vi "Read Cameras.vi"(8 "error in (no error)":errorcluster, 11 "Gantry Class in":refnum<class "Gantry Class.lvclass">) -> (0 "error out":errorcluster, 2 "Cameras":T1[](array[typedef]), 3 "Gantry Class out":refnum<class "Gantry Class.lvclass">)   [LabVIEW 2011, in "Gantry Class.lvclass"]
uses:
  Gantry Class.lvclass
  Type Definitions/Gantry_Camera.ctl
  <vilib>/userDefined/High Color/IMAQdx.ctl
  Gantry Class.lvclass/Gantry Class.ctl
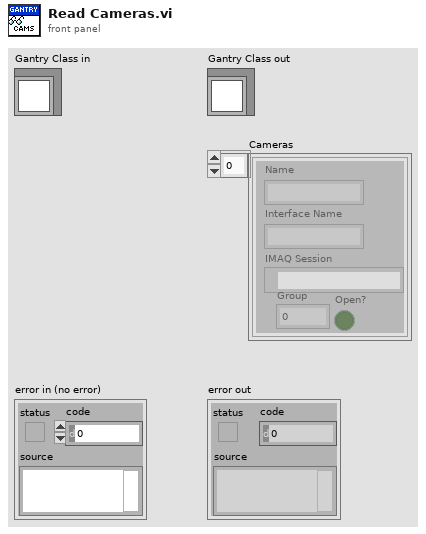
[diagram p1: front panel]
types:
  T1 = typedef "Gantry_Camera.ctl" = cluster{"Name":string, "IMAQ Session":T2, "Group":u32, "Open?":bool, "Interface Name":string}
  T2 = typedef "IMAQdx.ctl" = refnum<k21>
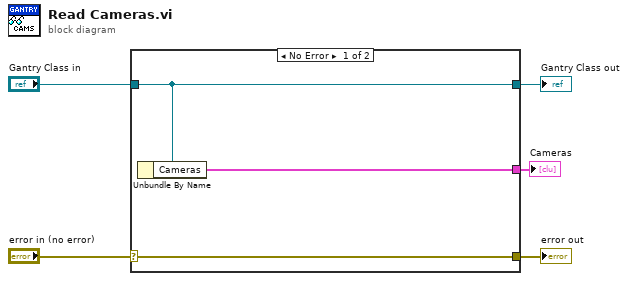
[diagram p0: block diagram]
diagram:
  n1 = case shown="No Error" "error in (no error)" {
    selector: "error in (no error)" -> [w8 w9]
    tunnel: [w8 w9] -> w4
    tunnel: [w7 w10] -> w2
    tunnel: "Gantry Class in" -> [w7 w10]
    tunnel: [w6 _] -> w1
    frame No Error {
      n2 = Unbundle By Name(w7) -> ("Cameras"=w6:T1[])
    }
    frame Error {
    }
  }
  "error out" <- w4
  "Gantry Class out" <- w2
  "Cameras" <- w1
